vi "CombineQueueText.vi"(2 "Queue in":string, 3 "Old List":string) -> (1 "New List":string)   [LabVIEW 2012]
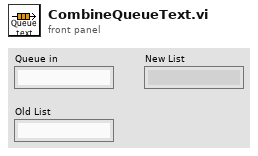
[diagram p1: front panel]
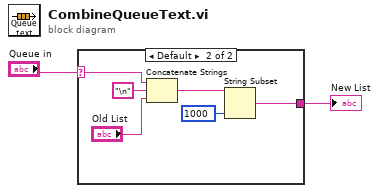
[diagram p0: block diagram]
diagram:
  n1 = case shown="Default" "Queue in" {
    selector: "Queue in" -> [w3 w4]
    tunnel: [w3 w6] -> w2
    frame "\u0000" {
    }
    frame Default {
      n2 = Concatenate Strings(w4, "\n" ("string"), "Old List") -> (w7:string)
      n3 = String Subset(string=w7, length (rest)=1000 ("length (rest)")) -> (substring=w6:string)  [unwired: 1 in]
    }
  }
  "New List" <- w2
